vi "Start.vi"(8 "error in (no error)":errorcluster, 11 "LV Chat Server in":refnum<class "LV Chat Server.lvclass">) -> (0 "error out":errorcluster, 3 "LV Chat Server out":refnum<class "LV Chat Server.lvclass">)   [LabVIEW 2020, in "LV Chat Server.lvclass"]
uses:
  LV Chat Server.lvclass
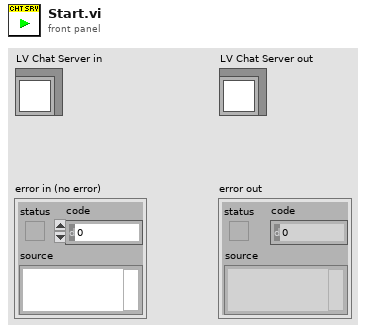
[diagram p1: front panel]
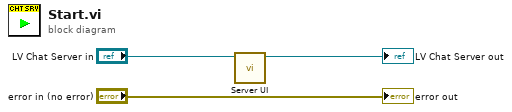
[diagram p0: block diagram]
diagram:
  n1 = call "Server UI.vi"("LV Chat Server in"="LV Chat Server in") -> ("LV Chat Server"=→"LV Chat Server out":refnum<class "LV Chat Server.lvclass">)  [unwired: 10 in]
  "error out" <- "error in (no error)"
